vi "CD Init_Prepare Inline Data_Fill In RT part of Frame Descriptor.vi"(8 "RTs In":T1[](array[typedef]) {"Mode Codes"."Words Item Refs" format="%.0x"; "Mode Codes"."Words Block Data Refs"."Data Reference" format="%.0x"; "Mode Codes"."Timestamp Channel Data Reference" format="%.0x"; "subAddresses"."Words Item Refs" format="%.0x"; "subAddresses"."Words Block Data Refs"."Data Reference" format="%.0x"; "subAddresses"."Timestamp Channel Data Reference" format="%.0x"; "Status Channel Data Reference" format="%.0x"; "Command Channels Refs" format="%.0x"}, 11 "message":T10 {"Timestamp Channel Data Reference" format="%.0x"; "Status Channel Data Refs" format="%.0x"; "Words Item Refs" format="%.0x"; "Words Block Data Refs"."Data Reference" format="%.0x"}) -> (0 "RTs Out":T1[](array[typedef]) {"Mode Codes"."Words Item Refs" format="%.0x"; "Mode Codes"."Words Block Data Refs"."Data Reference" format="%.0x"; "Mode Codes"."Timestamp Channel Data Reference" format="%.0x"; "subAddresses"."Words Item Refs" format="%.0x"; "subAddresses"."Words Block Data Refs"."Data Reference" format="%.0x"; "subAddresses"."Timestamp Channel Data Reference" format="%.0x"; "Status Channel Data Reference" format="%.0x"; "Command Channels Refs" format="%.0x"}, 3 "RT Frame Descriptor":T9 {"Status Channel Ref" format="%.0x"; "Words Block Data Refs"."Data Reference" format="%.0x"; "Timestamp Channel Data Reference" format="%.0x"})   [LabVIEW 2017, in "Ballard MIL-1553 Engine.lvlib"]
uses:
  Ballard MIL-1553 Engine.lvlib
  Shared/Controls and Global/RT Message.ctl
  Shared/Controls and Global/RT messageType.ctl
  Shared/Controls and Global/RT CWD1.ctl
  Shared/Controls and Global/RT CWD2.ctl
  <vilib>/NI Veristand/Custom Device API/Data Reference.ctl
  <vilib>/NI Veristand/Custom Device API/Custom Device Item Ref.ctl
  <vilib>/NI Veristand/Custom Device API/Block Data Reference.ctl
  Controls/RT Inline Frame Descriptor_RT.ctl
  Shared/Controls and Global/RT Remote Terminal.ctl
  Shared/Controls and Global/RT Remote Terminal_rtMode.ctl
  Shared/Controls and Global/RT Remote Terminal_RT subAddress.ctl
  Shared/Controls and Global/RT Remote Terminal_RT direction.ctl
  Shared/Controls and Global/RT Remote Terminal_RT Mode Code.ctl
  <vilib>/NI VeriStand/Custom Device API/Custom Device API.lvlib
  <vilib>/NI VeriStand/Custom Device Tools/Custom Device Utility Library/Custom Device Utility Library.lvlib
  Shared/Ballard 1553 Shared.lvlib
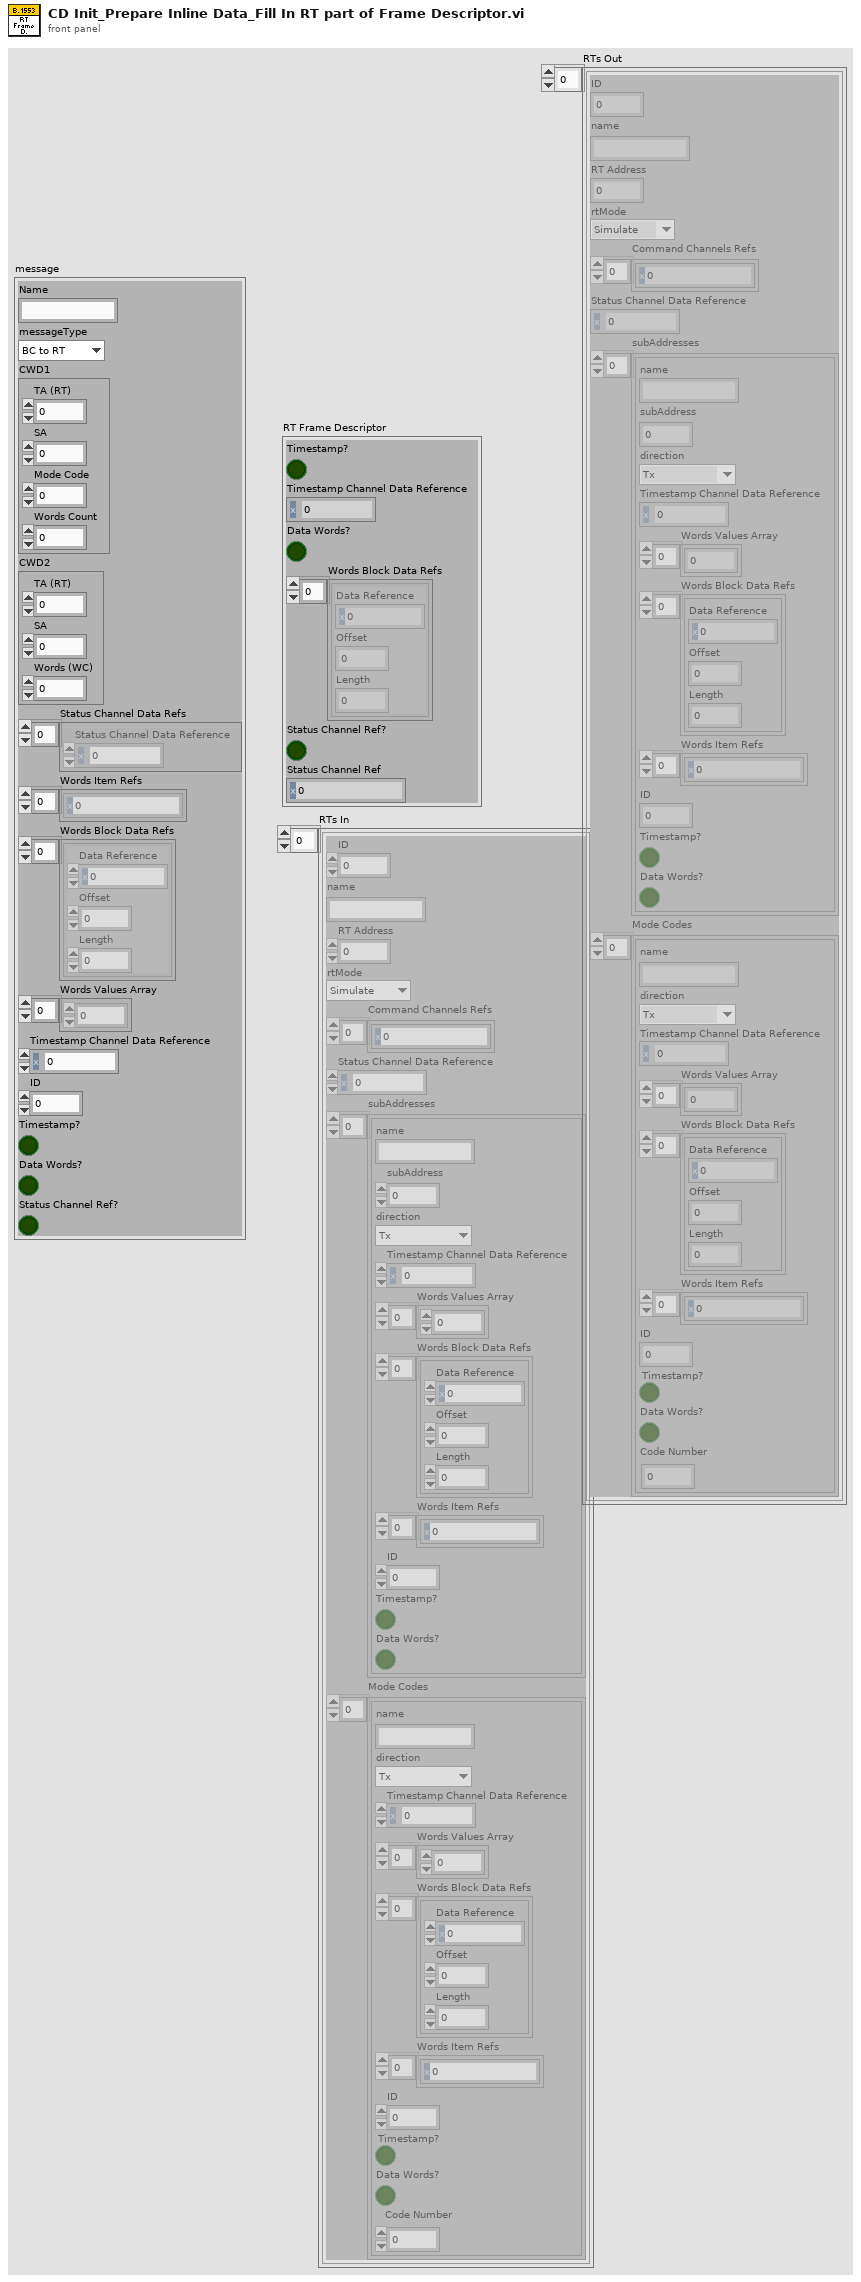
[diagram p1: front panel]
types:
  T1 = typedef "Ballard 1553 Shared.lvlib/RT Remote Terminal.ctl" = cluster{"ID":i32, "name":string, "RT Address":i32, "rtMode":T2, "Command Channels Refs":T3[], "Status Channel Data Reference":T4, "subAddresses":T5[], "Mode Codes":T8[]}
  T2 = typedef "Ballard 1553 Shared.lvlib/RT Remote Terminal_rtMode.ctl" = enum16{"Simulate", "Monitor", "Disable"}
  T3 = typedef "Custom Device API.lvlib/Custom Device Item Ref.ctl" = u64
  T4 = typedef "Custom Device API.lvlib/Data Reference.ctl" = i32
  T5 = typedef "Ballard 1553 Shared.lvlib/RT Remote Terminal_RT subAddress.ctl" = cluster{"name":string, "subAddress":i8, "direction":T6, "Timestamp Channel Data Reference":T4, "Words Values Array":u16[], "Words Block Data Refs":T7[], "Words Item Refs":T3[], "ID":i32, "Timestamp?":bool, "Data Words?":bool}
  T6 = typedef "Ballard 1553 Shared.lvlib/RT Remote Terminal_RT direction.ctl" = enum16{"Tx", "Rx"}
  T7 = typedef "Custom Device API.lvlib/Block Data Reference.ctl" = cluster{"Data Reference":T4, "Offset":u64, "Length":u64}
  T8 = typedef "Ballard 1553 Shared.lvlib/RT Remote Terminal_RT Mode Code.ctl" = cluster{"name":string, "direction":T6, "Timestamp Channel Data Reference":T4, "Words Values Array":u16[], "Words Block Data Refs":T7[], "Words Item Refs":T3[], "ID":i32, "Timestamp?":bool, "Data Words?":bool, "Code Number":i32}
  T9 = typedef "Ballard MIL-1553 Engine.lvlib/RT Inline Frame Descriptor_RT.ctl" = cluster{"Timestamp?":bool, "Timestamp Channel Data Reference":T4, "Data Words?":bool, "Words Block Data Refs":T7[], "Status Channel Ref?":bool, "Status Channel Ref":T3}
  T10 = typedef "Ballard 1553 Shared.lvlib/RT Message.ctl" = cluster{"Name":string, "messageType":T11, "CWD1":T12, "CWD2":T13, "Status Channel Data Refs":T4[], "Words Item Refs":T3[], "Words Block Data Refs":T7[], "Words Values Array":u16[], "Timestamp Channel Data Reference":T4, "ID":i32, "Timestamp?":bool, "Data Words?":bool, "Status Channel Ref?":bool}
  T11 = typedef "Ballard 1553 Shared.lvlib/RT messageType.ctl" = enum16{"BC to RT", "RT to BC", "RT to RT", "MC (Rx)", "MC (Tx)"}
  T12 = typedef "Ballard 1553 Shared.lvlib/RT CWD1.ctl" = cluster{"TA (RT)":i8, "SA":i8, "Mode Code":i8, "Words Count":i8}
  T13 = typedef "Ballard 1553 Shared.lvlib/RT CWD2.ctl" = cluster{"TA (RT)":i8, "SA":i8, "Words (WC)":i8}
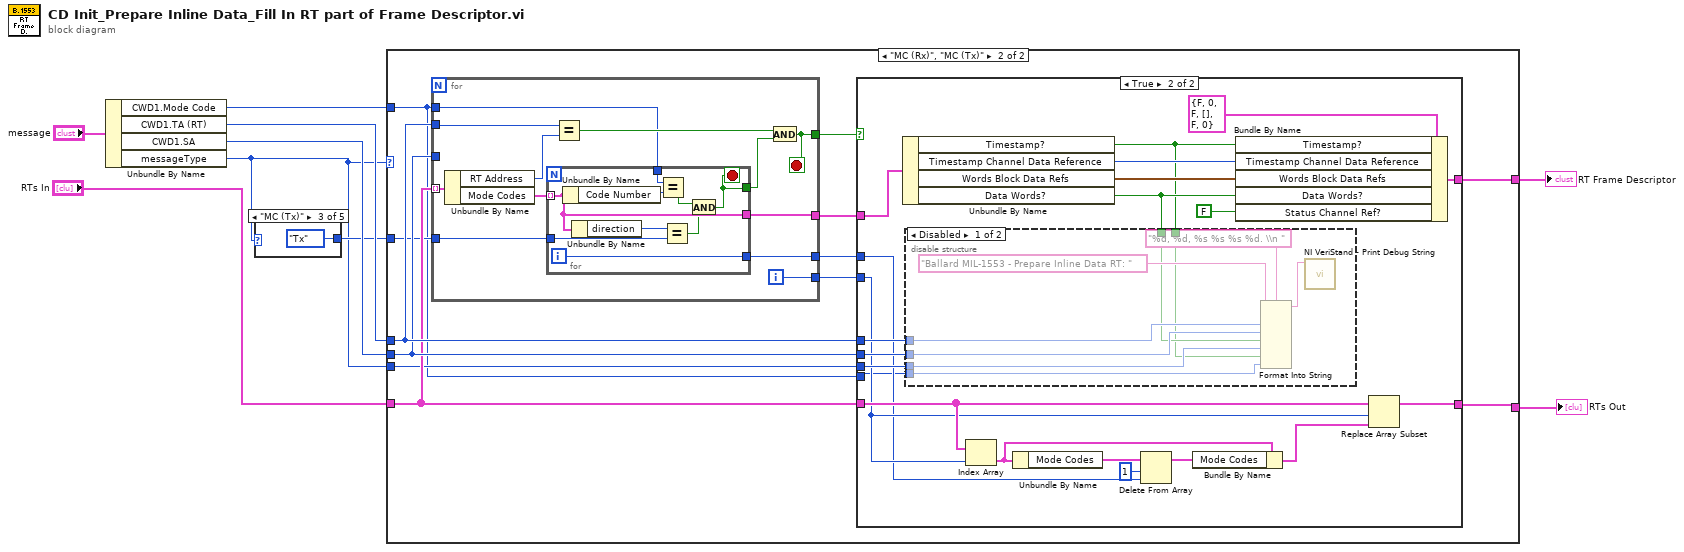
[diagram p0: block diagram]
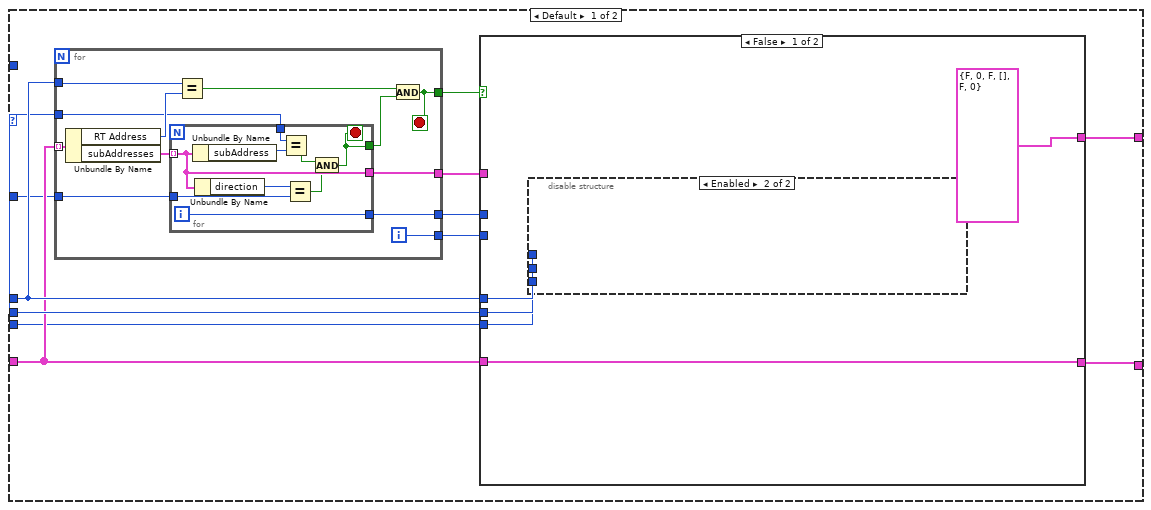
[diagram p2: hidden frame]
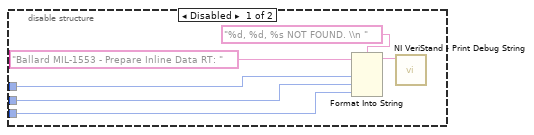
[diagram p3: hidden frame]
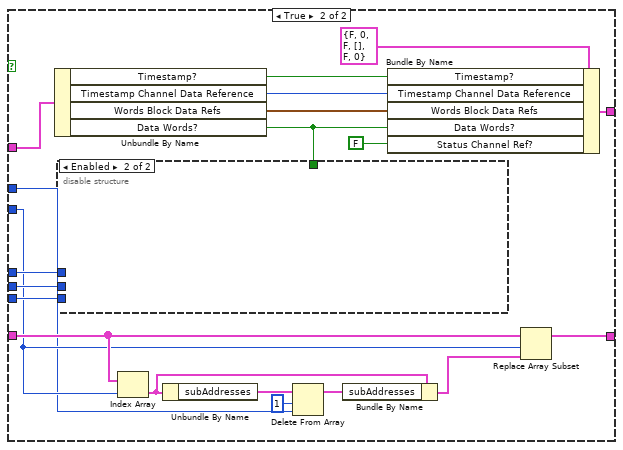
[diagram p4: hidden frame]
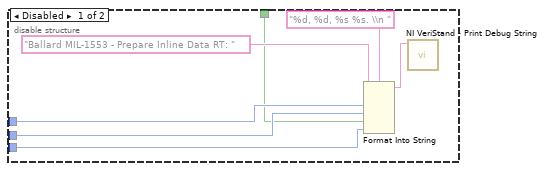
[diagram p5: hidden frame]
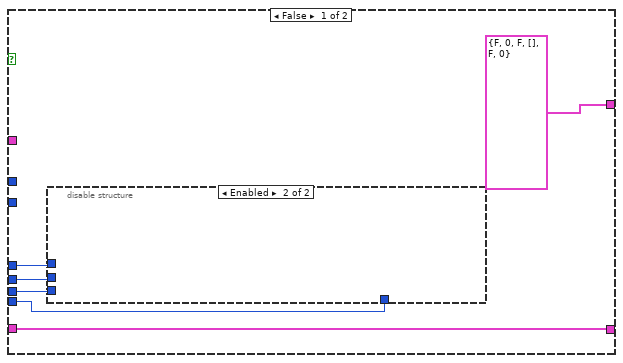
[diagram p6: hidden frame]
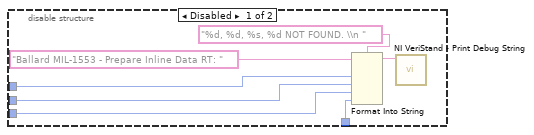
[diagram p7: hidden frame]
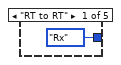
[diagram p9: hidden frame]
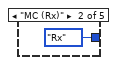
[diagram p10: hidden frame]
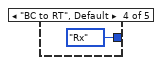
[diagram p11: hidden frame]
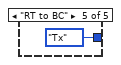
[diagram p12: hidden frame]
diagram:
  n1 = Unbundle By Name("message") -> ("CWD1.Mode Code"=w1:i8, "CWD1.TA (RT)"=w8:i8, "CWD1.SA"=w7:i8, "messageType"=w2:T11)
  n2 = case shown="\"MC (Tx)\"" w2 {
    tunnel: [RT_Remote_Terminal_RT_direction."Rx" ("y") RT_Remote_Terminal_RT_direction."Rx" ("y") RT_Remote_Terminal_RT_direction."Tx" ("y") RT_Remote_Terminal_RT_direction."Rx" ("y") RT_Remote_Terminal_RT_direction."Tx" ("y")] -> w3
    frame "RT to RT" {
    }
    frame "MC (Rx)" {
    }
    frame "MC (Tx)" {
    }
    frame "BC to RT", Default {
    }
    frame "RT to BC" {
    }
  }
  n3 = case shown="\"MC (Rx)\", \"MC (Tx)\"" w2 {
    tunnel: [w25 w96] -> w9
    tunnel: w8 -> [w22 w93]
    tunnel: w7 -> [w21 w92]
    tunnel: "RTs In" -> [w20 w91]
    tunnel: [w19 w90] -> w4
    tunnel: w3 -> [w18 w89]
    tunnel: w2 -> [w15 w86]
    tunnel: w1 -> [_ w85]
    frame Default {
      n4 = for {
        tunnel: w22 -> [w37]
        tunnel: w21 -> [w31]
        tunnel: w20 -> [w33] mode=indexing
        tunnel: [w34] -> w24
        tunnel: [w29] -> w23
        tunnel: w18 -> [w28]
        tunnel: [w27] -> w16
        tunnel: [w26] -> w17
        i -> [w26]
        stop <- w34 stop-if-true
        n5 = Unbundle By Name(w33) -> ("RT Address"=w36:i32, "subAddresses"=w32:T5[])
        n6 = for {
          tunnel: w32 -> [w44] mode=indexing
          tunnel: w31 -> [w46]
          tunnel: [w40] -> w30
          tunnel: [w44] -> w29
          tunnel: w28 -> [w39]
          tunnel: [w38] -> w27
          i -> [w38]
          stop <- w40 stop-if-true
          n7 = Unbundle By Name(w44) -> ("subAddress"=w45:i8)
          n8 = Unbundle By Name(w44) -> ("direction"=w43:T6)
          n9 = Equal?(x=w46, y=w45) -> (x = y?=w42:bool)
          n10 = Equal?(x=w43, y=w39) -> (x = y?=w41:bool)
          n11 = And(x=w42, y=w41) -> (x .and. y?=w40:bool)
        }
        n12 = Equal?(x=w37, y=w36) -> (x = y?=w35:bool)
        n13 = And(x=w35, y=w30) -> (x .and. y?=w34:bool)
      }
      n14 = case shown="False" w24 {
        tunnel: [T9 {"Timestamp?"=FALSE, "Timestamp Channel Data Reference"=0, "Data Words?"=FALSE, "Words Block Data Refs"=[], "Status Channel Ref?"=FALSE, "Status Channel Ref"=0} ("RT") w75] -> w25
        tunnel: w23 -> [_ w74]
        tunnel: w22 -> [w50 w72]
        tunnel: w21 -> [w49 w71]
        tunnel: w15 -> [w48 w67]
        tunnel: w20 -> [w47 w66]
        tunnel: [w47 w58] -> w19
        tunnel: w17 -> [_ w65]
        tunnel: w16 -> [_ w62]
        frame False {
          n15 = disable-structure shown="Enabled" {
            disable-tunnel: w50 -> [w54 _]
            disable-tunnel: w49 -> [w53 _]
            disable-tunnel: w48 -> [w52 _]
            frame Disabled {
              n16 = Format Into String(format string="%d, %d, %s NOT FOUND. \\n ", initial string="Ballard MIL-1553 - Prepare Inline Data RT: ", w54, w53, w52) -> (resulting string=w57:string)  [unwired: 1 in, 1 out]
              n17 = call <vilib>:"NI VeriStand - Print Debug String.vi"("Message"=w57) -> ()  [unwired: 10 in, 1 out]
            }
            frame Enabled {
            }
          }
        }
        frame True {
          n18 = Unbundle By Name(w74) -> ("Timestamp?"=w70:bool, "Timestamp Channel Data Reference"=w69:T4, "Words Block Data Refs"=w77:T7[], "Data Words?"=w68:bool)
          n19 = disable-structure shown="Enabled" {
            disable-tunnel: w72 -> [w83 _]
            disable-tunnel: w71 -> [w81 _]
            disable-tunnel: w68 -> [w79 _]
            disable-tunnel: w67 -> [w78 _]
            frame Disabled {
              n20 = Format Into String(format string="%d, %d, %s %s. \\n ", initial string="Ballard MIL-1553 - Prepare Inline Data RT: ", w83, w81, w79, w78) -> (resulting string=w80:string)  [unwired: 1 in, 1 out]
              n21 = call <vilib>:"NI VeriStand - Print Debug String.vi"("Message"=w80) -> ()  [unwired: 10 in, 1 out]
            }
            frame Enabled {
            }
          }
          n22 = Index Array(array=w66, index=w65) -> (element=w61:T1)
          n23 = Unbundle By Name(w61) -> ("subAddresses"=w64:T5[])
          n24 = Delete From Array(array=w64, length=1, index=w62) -> (array with subset deleted=w60:T5[])  [unwired: 1 out]
          n25 = Bundle By Name(cluster=w61, "subAddresses"=w60) -> (w59:T1)
          n26 = Bundle By Name(cluster=T9 {"Timestamp?"=FALSE, "Timestamp Channel Data Reference"=0, "Data Words?"=FALSE, "Words Block Data Refs"=[], "Status Channel Ref?"=FALSE, "Status Channel Ref"=0} ("RT"), "Timestamp?"=w70, "Timestamp Channel Data Reference"=w69, "Words Block Data Refs"=w77, "Data Words?"=w68, "Status Channel Ref?"=FALSE) -> (w75:T9)
          n27 = Replace Array Subset(array=w66, new element=w59, index=w65) -> (w58:T1[])
        }
      }
    }
    frame "MC (Rx)", "MC (Tx)" {
      n28 = for {
        tunnel: w93 -> [w108]
        tunnel: w92 -> [_]
        tunnel: w91 -> [w104] mode=indexing
        tunnel: [w105] -> w95
        tunnel: [w101] -> w94
        tunnel: w89 -> [w100]
        tunnel: [w99] -> w87
        tunnel: [w98] -> w88
        tunnel: w85 -> [w97]
        i -> [w98]
        stop <- w105 stop-if-true
        n29 = Unbundle By Name(w104) -> ("RT Address"=w107:i32, "Mode Codes"=w103:T8[])
        n30 = for {
          tunnel: w103 -> [w115] mode=indexing
          tunnel: w97 -> [w117]
          tunnel: [w111] -> w102
          tunnel: [w115] -> w101
          tunnel: w100 -> [w110]
          tunnel: [w109] -> w99
          i -> [w109]
          stop <- w111 stop-if-true
          n31 = Unbundle By Name(w115) -> ("Code Number"=w116:i32)
          n32 = Unbundle By Name(w115) -> ("direction"=w114:T6)
          n33 = Equal?(x=w117, y=w116) -> (x = y?=w113:bool)
          n34 = Equal?(x=w114, y=w110) -> (x = y?=w112:bool)
          n35 = And(x=w113, y=w112) -> (x .and. y?=w111:bool)
        }
        n36 = Equal?(x=w108, y=w107) -> (x = y?=w106:bool)
        n37 = And(x=w106, y=w102) -> (x .and. y?=w105:bool)
      }
      n38 = case shown="True" w95 {
        tunnel: [T9 {"Timestamp?"=FALSE, "Timestamp Channel Data Reference"=0, "Data Words?"=FALSE, "Words Block Data Refs"=[], "Status Channel Ref?"=FALSE, "Status Channel Ref"=0} ("RT") w149] -> w96
        tunnel: w94 -> [_ w148]
        tunnel: w93 -> [w122 w146]
        tunnel: w92 -> [w121 w145]
        tunnel: w86 -> [w120 w142]
        tunnel: w91 -> [w119 w141]
        tunnel: [w119 w133] -> w90
        tunnel: w88 -> [_ w140]
        tunnel: w87 -> [_ w137]
        tunnel: w85 -> [w118 w131]
        frame False {
          n39 = disable-structure shown="Enabled" {
            disable-tunnel: w122 -> [w127 _]
            disable-tunnel: w121 -> [w126 _]
            disable-tunnel: w120 -> [w125 _]
            disable-tunnel: w118 -> [w124 _]
            frame Disabled {
              n40 = Format Into String(format string="%d, %d, %s, %d NOT FOUND. \\n ", initial string="Ballard MIL-1553 - Prepare Inline Data RT: ", w127, w126, w125, w124) -> (resulting string=w130:string)  [unwired: 1 in, 1 out]
              n41 = call <vilib>:"NI VeriStand - Print Debug String.vi"("Message"=w130) -> ()  [unwired: 10 in, 1 out]
            }
            frame Enabled {
            }
          }
        }
        frame True {
          n42 = Unbundle By Name(w148) -> ("Timestamp?"=w132:bool, "Timestamp Channel Data Reference"=w144:T4, "Words Block Data Refs"=w151:T7[], "Data Words?"=w143:bool)
          n43 = disable-structure shown="Disabled" {
            disable-tunnel: w146 -> [w159 _]
            disable-tunnel: w145 -> [w157 _]
            disable-tunnel: w143 -> [w155 _]
            disable-tunnel: w142 -> [w154 _]
            disable-tunnel: w132 -> [w153 _]
            disable-tunnel: w131 -> [w152 _]
            frame Disabled {
              n44 = Format Into String(format string="%d, %d, %s %s %s %d. \\n ", initial string="Ballard MIL-1553 - Prepare Inline Data RT: ", w159, w157, w155, w154, w153, w152) -> (resulting string=w156:string)  [unwired: 1 in, 1 out]
              n45 = call <vilib>:"NI VeriStand - Print Debug String.vi"("Message"=w156) -> ()  [unwired: 10 in, 1 out]
            }
            frame Enabled {
            }
          }
          n46 = Index Array(array=w141, index=w140) -> (element=w136:T1)
          n47 = Unbundle By Name(w136) -> ("Mode Codes"=w139:T8[])
          n48 = Delete From Array(array=w139, length=1, index=w137) -> (array with subset deleted=w135:T8[])  [unwired: 1 out]
          n49 = Bundle By Name(cluster=w136, "Mode Codes"=w135) -> (w134:T1)
          n50 = Bundle By Name(cluster=T9 {"Timestamp?"=FALSE, "Timestamp Channel Data Reference"=0, "Data Words?"=FALSE, "Words Block Data Refs"=[], "Status Channel Ref?"=FALSE, "Status Channel Ref"=0} ("RT"), "Timestamp?"=w132, "Timestamp Channel Data Reference"=w144, "Words Block Data Refs"=w151, "Data Words?"=w143, "Status Channel Ref?"=FALSE) -> (w149:T9)
          n51 = Replace Array Subset(array=w141, new element=w134, index=w140) -> (w133:T1[])
        }
      }
    }
  }
  "RT Frame Descriptor" <- w9
  "RTs Out" <- w4
